vi "PostControlPanelRefnum.vi"(8 "error in (no error)":errorcluster, 9 "VI Refnum":refnum<vi>, 10 "Panel":string, 11 "DockingDevice in":refnum<class "DockingDevice.lvclass">) -> (0 "error out":errorcluster, 3 "DockingDevice out":refnum<class "DockingDevice.lvclass">)   [LabVIEW 2020, in "DockingDevice.lvclass"]
uses:
  DockingDevice.lvclass
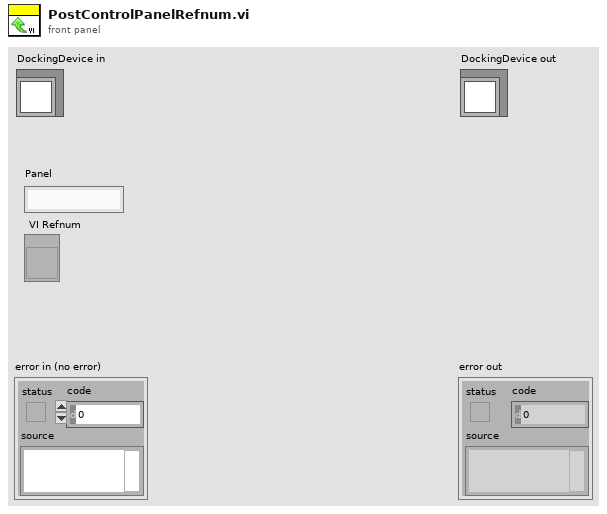
[diagram p1: front panel]
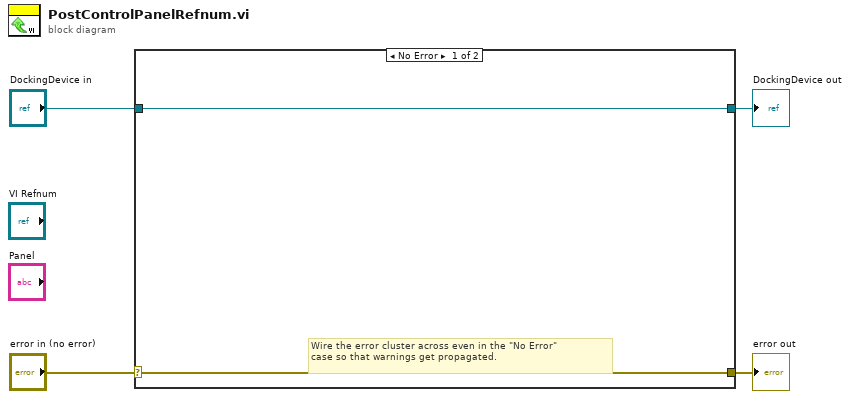
[diagram p0: block diagram]
diagram:
  n1 = case shown="No Error" "error in (no error)" {
    selector: "error in (no error)" -> [w5 w8]
    tunnel: [w5 w8] -> w3
    tunnel: [w6 w7] -> w1
    tunnel: "DockingDevice in" -> [w6 w7]
    frame No Error {
      # "Wire the error cluster across even in the \"No Error\"\ncase so that warnings get propagated."
    }
    frame Error {
    }
  }
  "error out" <- w3
  "DockingDevice out" <- w1
